vi "Qrcode 2D Array testing.vi"() -> ()   [LabVIEW 2019]
uses:
  <vilib>/userDefined/High Color/IMAQdx.ctl
  <vilib>/vision/driver/NI_Vision_Acquisition_Software.lvlib
  <vilib>/vision/NI_Vision_Development_Module.lvlib
panel:
  in  "ROI Descriptor":T1 {"Contours"."Type" items=["No Selection", "Point", "Line", "Rectangle", "Oval", "Polygon", "Freehand Region", "Annulus", "Unused2", "Unused3", "Broken Line", "Freehand Line", "Rotated Rectangle"]}
  in  "Session In":T2
  out "Image":T3(plugin-control)
  out "Found ?":bool
  out "Data":string
  in  "new element/subarray 2":string
  in  "col":i32
  in  "index":i32
  in  "Array":string[][](array[string])=[["invalid", "invalid", "invalid"], ["invalid", "invalid", "invalid"], ["invalid", "invalid", "invalid"]]
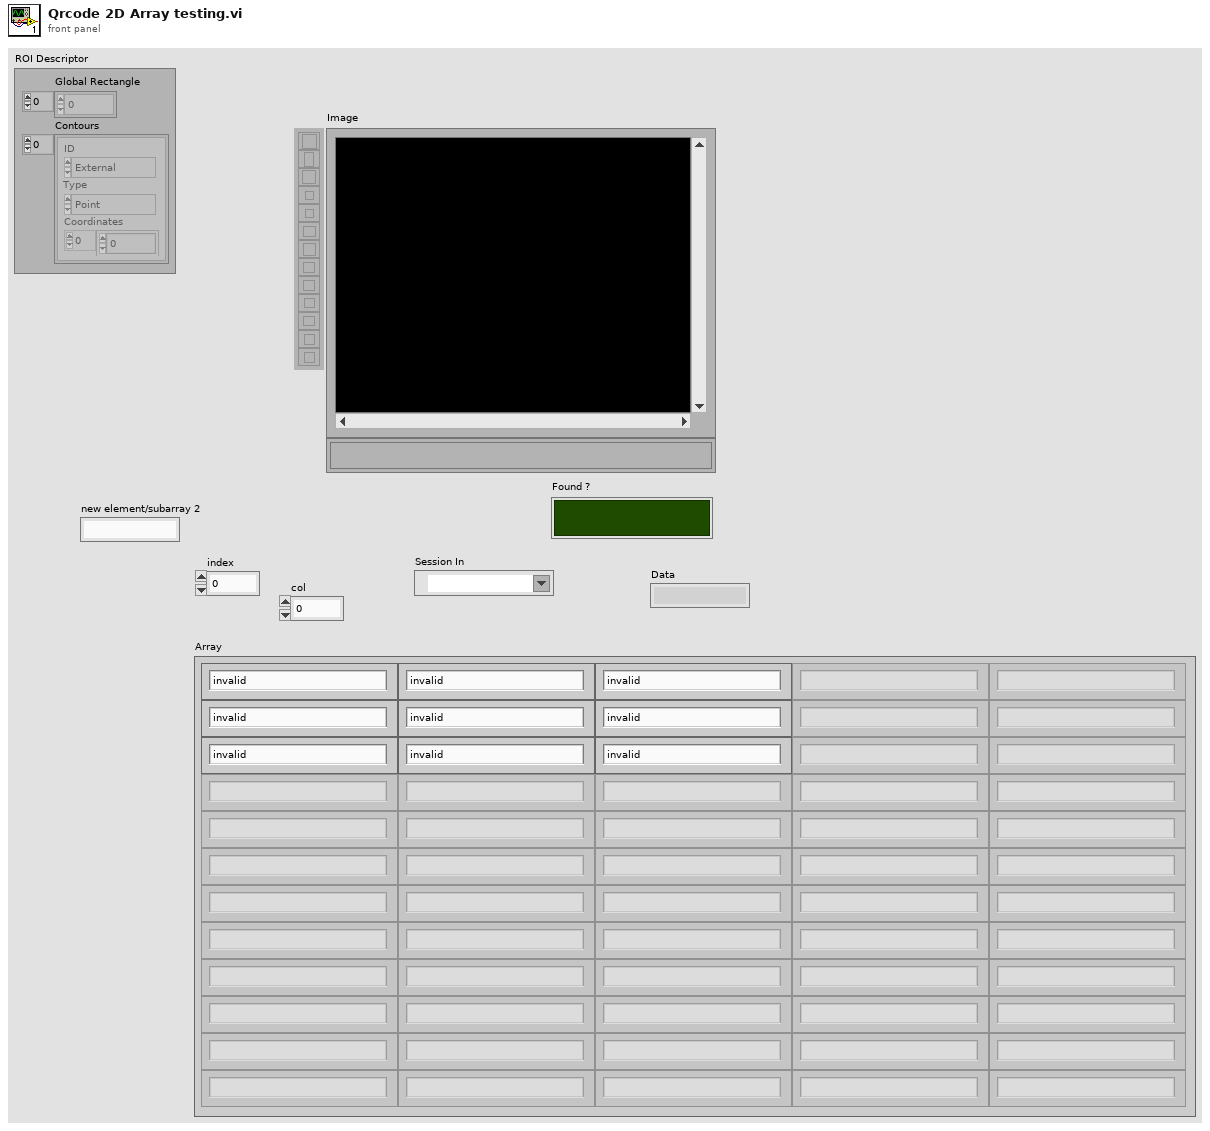
[diagram p1: front panel]
types:
  T1 = typedef "ROI Descriptor" = cluster{"Global Rectangle":i32[], "Contours":cluster{"ID":enum32{"External", "Internal"}, "Type":u32, "Coordinates":i32[]}[]}
  T2 = typedef "IMAQdx.ctl" = refnum<k21>
  T3 = typedef "IMAQ Image.ctl" = refnum<image>
  T4 = enum16{"qrcode scan", "check 1", "insert", "increament", "check 2", "stop"}
  T5 = typedef "QR Code Report.ctl" = cluster{"Found?":bool, "Data":string, "Bounding Box":cluster{"x":sgl, "y":sgl}[], "Errors Corrected":u32, "Dimensions (Rows/Cols)":u32, "Version":u32, "QR Model":T6, "Stream Mode":T7, "Barcode Polarity":T8, "Mirrored?":bool, "Append Stream Position":u32, "Size of Append Stream":u32, "First EAN-128 ID":i32, "First Alternate Language ID":i32, "Append Stream ID":u32, "Minimum Edge Strength":u32, "Demodulation Mode":T9, "Cell Sample Size":T10, "Cell Filter Mode":T11}
  T6 = typedef "QR Code Model Type.ctl" = i32
  T7 = typedef "QR Code Stream Mode Type.ctl" = i32
  T8 = typedef "Data Matrix Polarity.ctl" = i32
  T9 = typedef "Demodulation Mode.ctl" = i32
  T10 = typedef "Cell Sample Size.ctl" = i32
  T11 = typedef "Cell Filter Mode.ctl" = i32
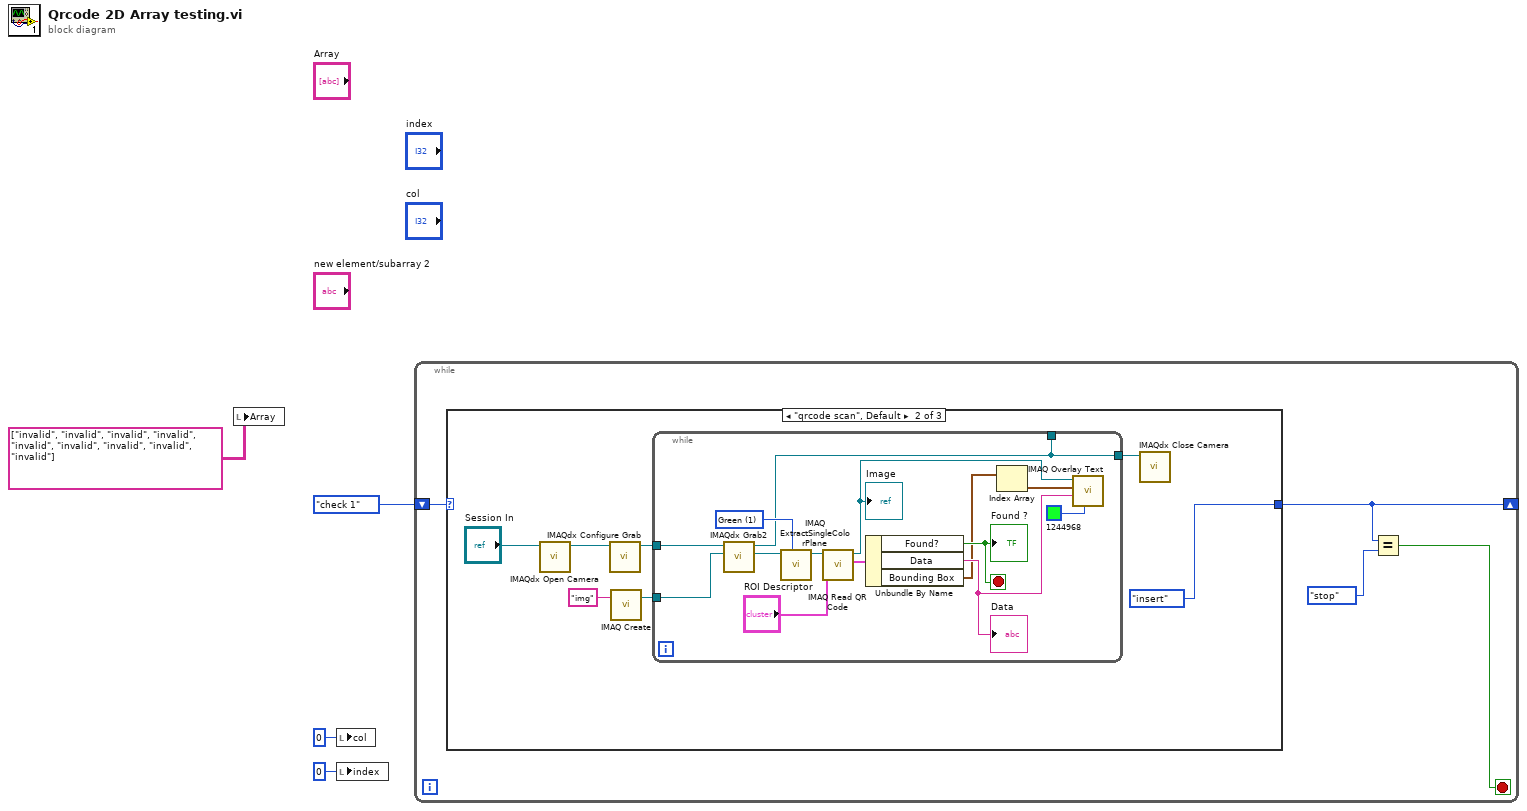
[diagram p0: block diagram]
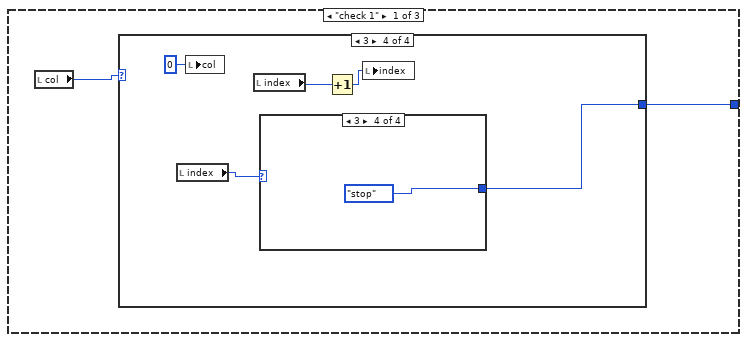
[diagram p2: hidden frame]
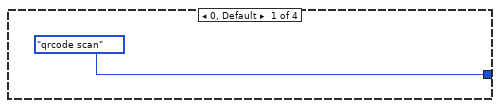
[diagram p3: hidden frame]
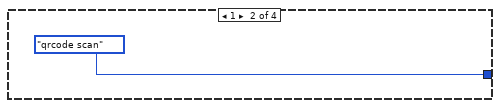
[diagram p4: hidden frame]
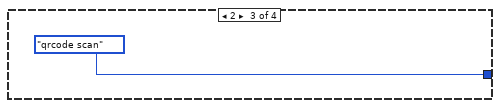
[diagram p5: hidden frame]
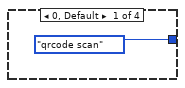
[diagram p6: hidden frame]
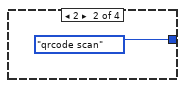
[diagram p7: hidden frame]
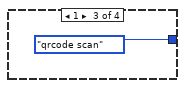
[diagram p8: hidden frame]
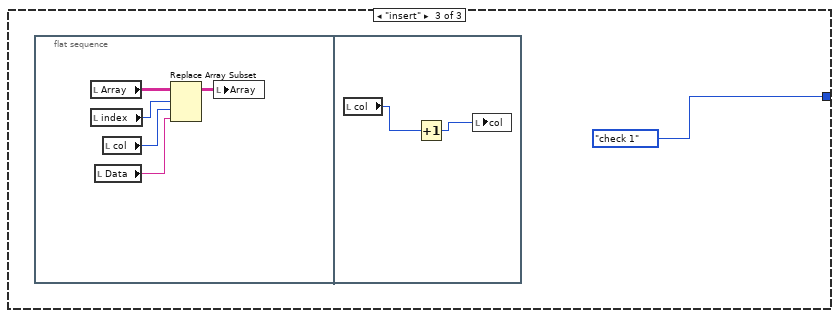
[diagram p9: hidden frame]
diagram:
  n1 = local write "Array"(string[][] [["invalid", "invalid", "invalid"], ["invalid", "invalid", "invalid"], ["invalid", "invalid", "invalid"]] ("Array")) -> ()
  n2 = local write "col"(0 ("col")) -> ()
  n3 = local write "index"(0 ("index")) -> ()
  n4 = while {
    shift-right: [w6] -> _
    shift-left: T4."check 1" -> [w8]
    stop <- w5 stop-if-true
    n5 = case shown="\"qrcode scan\", Default" w8 {
      tunnel: [w9 T4."insert" T4."check 1"] -> w6
      frame "check 1" {
        n6 = local read "col"() -> (w10:i32)
        n7 = case shown="3" w10 {
          tunnel: [T4."qrcode scan" T4."qrcode scan" T4."qrcode scan" w14] -> w9
          frame 0, Default {
          }
          frame 1 {
          }
          frame 2 {
          }
          frame 3 {
            n8 = local read "index"() -> (w15:i32)
            n9 = local write "col"(0 ("col")) -> ()
            n10 = local read "index"() -> (w16:i32)
            n11 = case shown="3" w15 {
              tunnel: [T4."qrcode scan" T4."qrcode scan" T4."qrcode scan" T4."stop"] -> w14
              frame 0, Default {
              }
              frame 2 {
              }
              frame 1 {
              }
              frame 3 {
              }
            }
            n12 = Increment(x=w16) -> (x+1=w17:i32)
            n13 = local write "index"(w17) -> ()
          }
        }
      }
      frame "qrcode scan", Default {
        n14 = call <vilib>:"IMAQdx Open Camera.vi"("Session In"="Session In") -> ("Session Out"=w29:T2)  [unwired: 9 in, 1 out]
        n15 = call <vilib>:"IMAQdx Configure Grab.vi"("Session In"=w29) -> ("Session Out"=w28:T2)  [unwired: 9 in, 1 out]
        n16 = call "IMAQ Create"("Image Name"="img") -> ("New Image"=w25:T3)  [unwired: 4 in, 1 out]
        n17 = while {
          tunnel: w28 -> [w43]
          tunnel: [w30] -> w27
          tunnel: w25 -> [w40]
          tunnel: [w30] -> _
          stop <- w41 stop-if-true
          w39 = 1 items=["Red", "Green", "Blue", "Hue", "Saturation", "Luminance", "Value", "Intensity"] ("Color Plane")
          n18 = call <vilib>:"IMAQdx Grab2.vi"("Image In"=w40, "Session In"=w43) -> ("Image Out"=w32:T3, "Session Out"=w30:T2)  [unwired: 6 in, 2 out]
          n19 = call "IMAQ ExtractSingleColorPlane"("Color Plane"=w39, "Image Src"=w32) -> ("Image Dst Out"=w38:T3)  [unwired: 8 in, 1 out]
          n20 = call "IMAQ Read QR Code"("ROI Descriptor"="ROI Descriptor", "Image"=w38) -> ("QR Code Report"=w42:T5, "Image (duplicate)"=w34:T3)  [unwired: 6 in, 2 out]
          "Image" <- w34
          n21 = Unbundle By Name(w42) -> ("Found?"=w41:bool, "Data"=w36:string, "Bounding Box"=w33:cluster{"x":sgl, "y":sgl}[])
          "Found ?" <- w41
          "Data" <- w36
          n22 = Index Array(array=w33) -> (element=w37:cluster{"x":sgl, "y":sgl})  [unwired: 1 in]
          n23 = call "IMAQ Overlay Text"("Text Color (black)"=u32 1244968, "String"=w36, "Origin"=w37, "Image"=w34) -> ()  [unwired: 6 in, 2 out]
        }
        n24 = call <vilib>:"IMAQdx Close Camera.vi"("Session In"=w27) -> ()  [unwired: 10 in, 1 out]
      }
      frame "insert" {
        n25 = flat-sequence {
          frame #0 {
            n26 = local read "Array"() -> (w48:string[][])
            n27 = local read "index"() -> (w47:i32)
            n28 = local read "Data"() -> (w45:string)
            n29 = local read "col"() -> (w46:i32)
            n30 = Replace Array Subset(array=w48, new element=w45, index (row)=w47, index (col)=w46) -> (w49:string[][])
            n31 = local write "Array"(w49) -> ()
          }
          frame #1 {
            n32 = local read "col"() -> (w51:i32)
            n33 = Increment(x=w51) -> (x+1=w50:i32)
            n34 = local write "col"(w50) -> ()
          }
        }
      }
    }
    n35 = Equal?(x=w6, y=T4."stop") -> (x = y?=w5:bool)
  }
